vi "ActionVIOnSave (File).vi"(8 "error in":errorcluster, 11 "file item reference in":T1 format="%.0x") -> (0 "error out":errorcluster, 3 "file item reference out":T1 format="%.0x")   [LabVIEW 2019, in "Telemetry System Explorer.lvlib"]
uses:
  Telemetry System Explorer.lvlib
  <vilib>/NI VeriStand/Custom Device API/Custom Device Item Ref.ctl
  <vilib>/NI VeriStand/Custom Device API/Custom Device API.lvlib
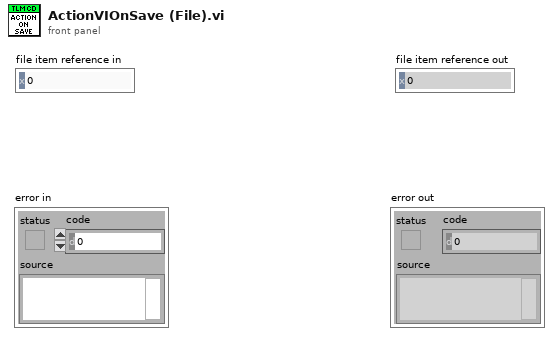
[diagram p1: front panel]
types:
  T1 = typedef "Custom Device API.lvlib/Custom Device Item Ref.ctl" = u64
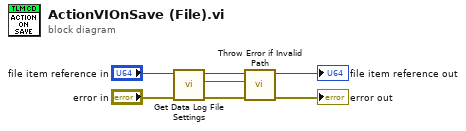
[diagram p0: block diagram]
diagram:
  n1 = call "Get Data Log File Settings.vi"("error in (no error)"="error in", "File Ref In"="file item reference in") -> ("error out"=w5:errorcluster, "File Path"=w4:path, "File Ref Out"=w3:T1)  [unwired: 5 in, 2 out]
  n2 = call "Throw Error if Invalid Path.vi"("error in"=w5, "file path"=w4, "item reference in"=w3) -> ("error out"=→"error out":errorcluster, "item reference out"=→"file item reference out":T1)  [unwired: 7 in]
